vi "Ramp Status.vi"(8 "error in (no error)":errorcluster, 10 "Output's Control Loop (1:1)":u16(ring)=1 items=["1"=1, "2"=2], 11 "VISA resource name":refnum<visa-resource-name>) -> (0 "error out":errorcluster, 1 "Ramping Active?":bool, 2 "Ramping On?":bool, 3 "VISA resource name out":refnum<visa-resource-name>, 5 "Ramp Rate":dbl format="%.1f")   [LabVIEW 2021, in "Lake Shore 336.lvlib"]
doc: "This VI returns the status of the setpoint ramp function. The Model 336 can generate a smooth setpoint ramp when the setpoint units are expressed in temperature. Once the ramping feature is turned on, its action is initiated by a setpoint change. When a new setpoint is entered, the instrument changes the setpoint temperature from the old value to the new value at the ramp rate. The Setpoint Ramping function applies to the Heater Outputs (1 and 2) only."
uses:
  <instrlib>/Lake Shore 336/Lake Shore 336.lvlib
  Instance           1 19Saved   Ramp Status .vi
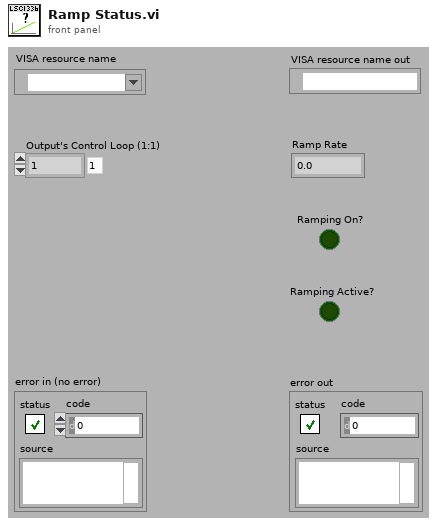
[diagram p1: front panel]
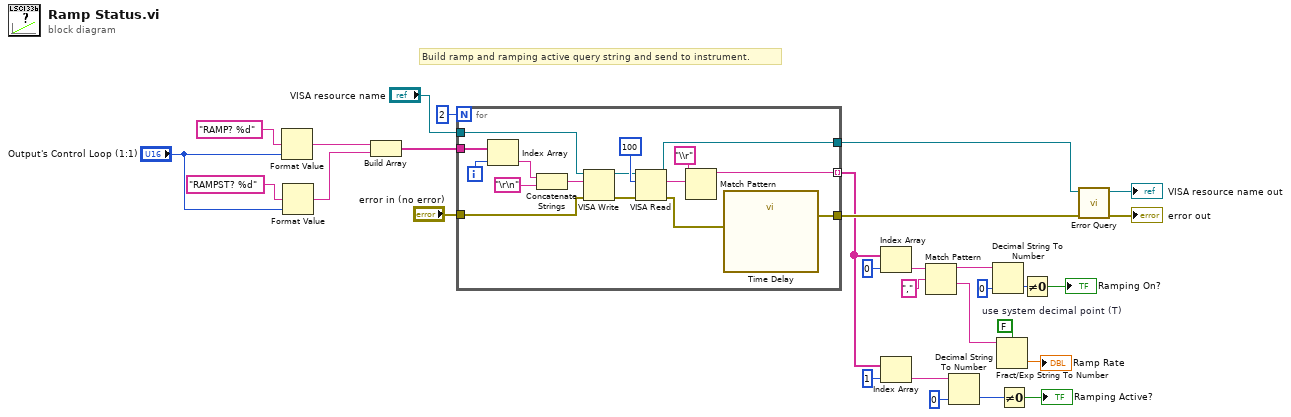
[diagram p0: block diagram]
diagram:
  w29 = FALSE  # use system decimal point (T)
  # "Build ramp and ramping active query string and send to instrument."
  n1 = Format Value(format string="RAMP? %d", value (0)="Output's Control Loop (1:1)") -> (output string=w3:string)  [unwired: 1 in]
  n2 = Format Value(format string="RAMPST? %d", value (0)="Output's Control Loop (1:1)") -> (output string=w2:string)  [unwired: 1 in]
  n3 = Build Array(w3, w2) -> (w22:string[])
  n4 = for {
    N: 2 -> [_]
    tunnel: [w39] -> w28
    tunnel: [w33] -> w27
    tunnel: "VISA resource name" -> [w38]
    tunnel: "error in (no error)" -> [w37]
    tunnel: w22 -> [w36]
    tunnel: [w35] -> w17 mode=indexing
    i -> [w40]
    n5 = Index Array(array=w36, index=w40) -> (element=w31:string)
    n6 = Concatenate Strings(w31, "\r\n") -> (w32:string)
    n7 = VISA Write(VISA resource name=w38, write buffer=w32, error in (no error)=w37) -> (VISA resource name out=w42:refnum<visa-resource-name>, error out=w41:errorcluster)  [unwired: 1 out]
    n8 = VISA Read(VISA resource name=w42, byte count=100, error in (no error)=w41) -> (VISA resource name out=w39:refnum<visa-resource-name>, read buffer=w44:string, error out=w34:errorcluster)  [unwired: 1 out]
    n9 = Match Pattern(string=w44, regular expression="\\r") -> (before substring=w35:string)  [unwired: 1 in, 3 out]
    n10 = call "Time Delay"("error in (no error)"=w34) -> ("error out"=w33:errorcluster)  [unwired: 10 in]
  }
  n11 = Index Array(array=w17, index=0) -> (element=w11:string)
  n12 = Index Array(array=w17, index=1) -> (element=w16:string)
  n13 = Match Pattern(string=w11, regular expression=",") -> (before substring=w6:string, after substring=w7:string)  [unwired: 1 in, 2 out]
  n14 = Decimal String To Number(string=w16, default (0L)=u16 0) -> (number=w9:u16)  [unwired: 1 in, 1 out]
  n15 = Decimal String To Number(string=w6, default (0L)=u16 0) -> (number=w12:u16)  [unwired: 1 in, 1 out]
  n16 = Fract/Exp String To Number(use system decimal point (T)=w29, string=w7) -> (number=→"Ramp Rate":dbl)  [unwired: 2 in, 1 out]
  n17 = Not Equal To 0?(x=w9) -> (x != 0?=→"Ramping Active?":bool)
  n18 = Not Equal To 0?(x=w12) -> (x != 0?=→"Ramping On?":bool)
  n19 = call <instrlib>:"Error Query.vi"("error in (no error)"=w27, "VISA resource name"=w28) -> ("error out"=→"error out":errorcluster, "VISA resource name out"=→"VISA resource name out":refnum<visa-resource-name>)  [unwired: 7 in, 1 out]
